vi "Combine Vectors.vi"(10 "Rotation Module Data":T1 {"Angle" scale format="%.3f"; "Velocity" scale=-1.0..1.0 scale format="%.1f"}, 11 "Travers Module Data":T1 {"Angle" scale format="%.3f"; "Velocity" scale=-1.0..1.0 scale format="%.1f"}) -> (2 "Velocity Out":dbl, 3 "Combine Out":T1 {"Angle" scale format="%.3f"; "Velocity" scale=-1.0..1.0 scale format="%.1f"})   [LabVIEW 2023, in "SwerveDrive_ACT_ts.lvlib"]
uses:
  SwerveDrive_ACT_ts.lvlib
  Shared Code/TypeDefs/Cluster_Module Velocity-Direction-Rotations.ctl
  Shared Code/TypeDefs/Level_Velocity plus-minus 1.ctl
  Shared Code/TypeDefs/Dial_Compase heading unit circle CCW positive.ctl
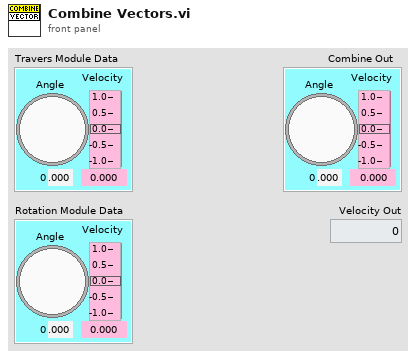
[diagram p1: front panel]
types:
  T1 = typedef "Cluster_Module Velocity-Direction-Rotations.ctl" = cluster{"Velocity":T2, "Angle":T3, "Rotations Count":dbl}
  T2 = typedef "Level_Velocity plus-minus 1.ctl" = dbl
  T3 = typedef "Dial_Compase heading unit circle CCW positive.ctl" = dbl
  T4 = typedef "Cluster_X-Y.ctl" = cluster{"X":dbl, "Y":dbl}
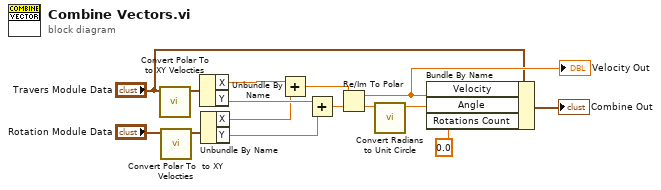
[diagram p0: block diagram]
diagram:
  n1 = call "Convert Polar To  to XY Velocties.vi"("Traverse"="Travers Module Data") -> ("XY Velocities Out"=w4:T4)  [unwired: 10 in]
  n2 = call "Convert Polar To  to XY Velocties.vi"("Traverse"="Rotation Module Data") -> ("XY Velocities Out"=w3:T4)  [unwired: 10 in]
  n3 = Unbundle By Name(w4) -> ("X"=w9:dbl, "Y"=w8:dbl)
  n4 = Unbundle By Name(w3) -> ("X"=w7:dbl, "Y"=w6:dbl)
  n5 = Add(x=w9, y=w7) -> (x+y=w14:dbl)
  n6 = Add(x=w8, y=w6) -> (x+y=w15:dbl)
  n7 = Re/Im To Polar(2:w15, 3:w14) -> (0:w13:dbl, 1:w10:dbl)
  "Velocity Out" <- w10
  n8 = call "Convert Radians to Unit Circle.vi"("Radians"=w13) -> ("Unit Circle"=w12:dbl)  [unwired: 10 in]
  n9 = Bundle By Name(cluster="Travers Module Data", "Velocity"=w10, "Angle"=w12, "Rotations Count"=0.0 ("Rotations")) -> (→"Combine Out":T1)
